vi "Finish.vi"(8 "error in (no error)":errorcluster, 11 "Elevator Concrete in":refnum<class "Elevator Arm.lvclass">) -> (0 "error out":errorcluster, 3 "Elevator Concrete out":refnum<class "Elevator Arm.lvclass">)   [LabVIEW 2019, in "Elevator.lvlib" / "Elevator Arm.lvclass"]
uses:
  Elevator Arm.lvclass
  Elevator.lvclass
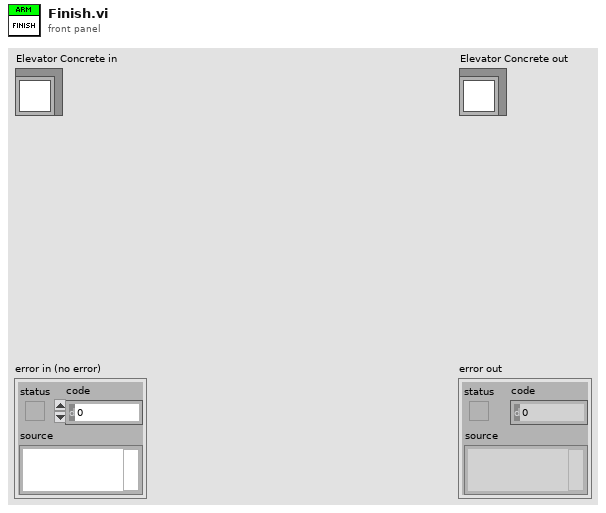
[diagram p1: front panel]
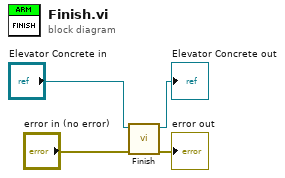
[diagram p0: block diagram]
diagram:
  n1 = call-parent "Finish.vi"("error in (no error)"="error in (no error)", "Elevator in"="Elevator Concrete in") -> ("error out"=→"error out":errorcluster, "Elevator out"=→"Elevator Concrete out":refnum<class "Elevator Arm.lvclass">)  [unwired: 8 in]
